vi "Mask Joysticks.vi"(6 "Operator POVs":i16[](array[numeric])=[-1], 7 "Driver Axes":dbl[](array[numeric]), 8 "Operator Buttons":bool[](array[boolean])=[FALSE, FALSE, FALSE, FALSE, FALSE, FALSE, FALSE, FALSE, FALSE, FALSE], 9 "Operator Axes":dbl[](array[numeric])=[0.0, -0.007874015748031496, 0.0, 0.0, 0.0, 0.0], 10 "Driver POVs":i16[](array[numeric]), 11 "Driver Buttons":bool[](array[boolean])=[TRUE, FALSE, FALSE, FALSE, FALSE, FALSE, FALSE, FALSE, FALSE, TRUE]) -> (0 "Operator Buttons Out":bool[](array[boolean]), 1 "Operator Axes Out":dbl[](array[numeric]), 2 "Driver POVs Out":i16[](array[numeric]), 3 "Drive Buttons Out":bool[](array[boolean])=[TRUE, FALSE, FALSE, FALSE, FALSE, FALSE, FALSE, FALSE, FALSE, TRUE], 4 "Operator POVs Out":i16[](array[numeric])=[-1], 5 "Drive Axes Out":dbl[](array[numeric]))   [LabVIEW 2018]
panel:
  out "Time to excecute ms":u32
  in  "Operator Axes Mask":bool[](array[boolean])=[TRUE, TRUE, TRUE, TRUE, TRUE, TRUE, TRUE, TRUE, TRUE, TRUE]
  in  "Operator Buttons Mask":bool[](array[boolean])=[TRUE, TRUE, TRUE, TRUE, TRUE, TRUE, TRUE, TRUE, TRUE, TRUE]
  in  "D315":bool
  in  "D270":bool
  in  "D235":bool
  in  "D135":bool
  in  "D180":bool
  in  "D90":bool
  in  "D45":bool
  in  "D0/360":bool
  in  "Driver Buttons Mask":bool[](array[boolean])=[TRUE, TRUE, TRUE, TRUE, TRUE, TRUE, TRUE, TRUE, TRUE, TRUE]
  in  "Driver Axes Mask":bool[](array[boolean])=[TRUE, TRUE, TRUE, TRUE, TRUE, TRUE, TRUE, TRUE, TRUE, TRUE]
  # "POV Mask"
  # "POV Masking Not DOne"
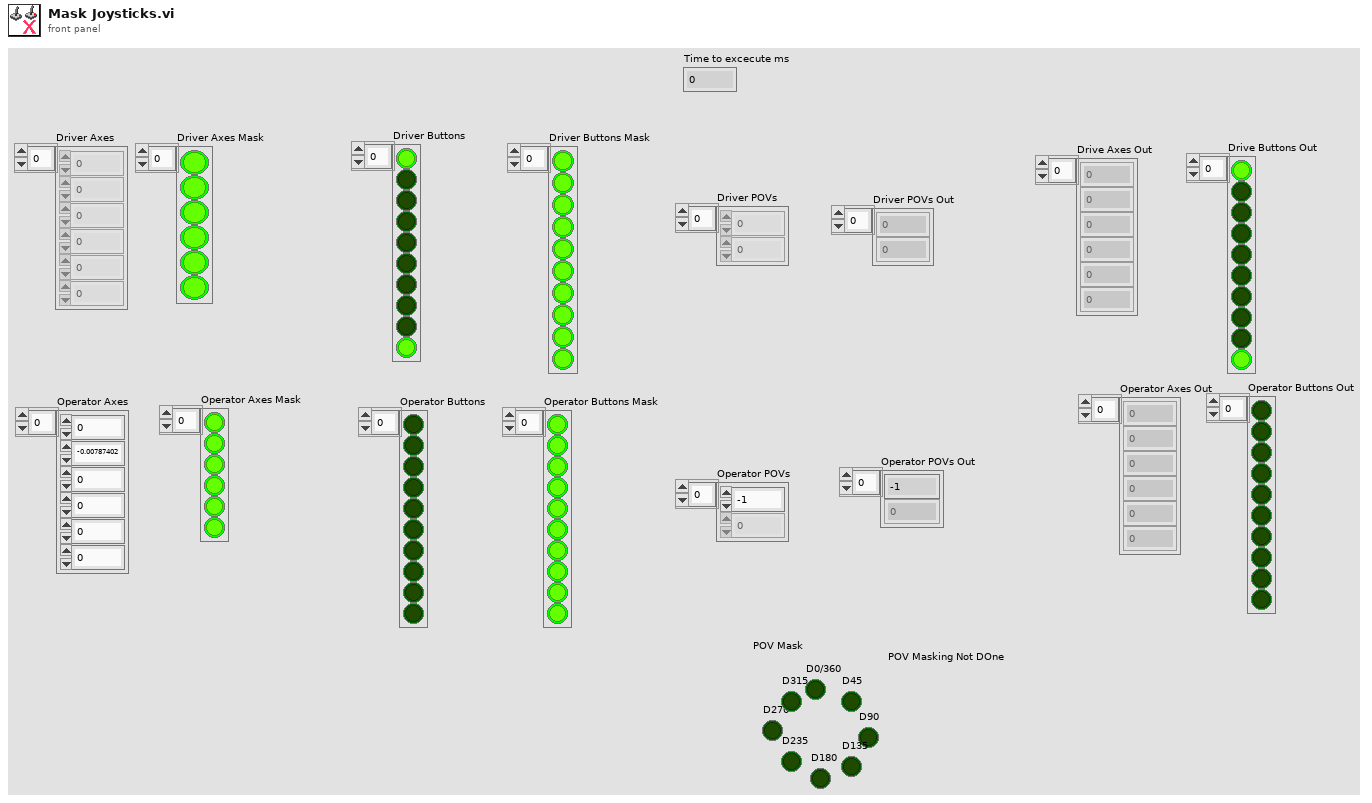
[diagram p1: front panel]
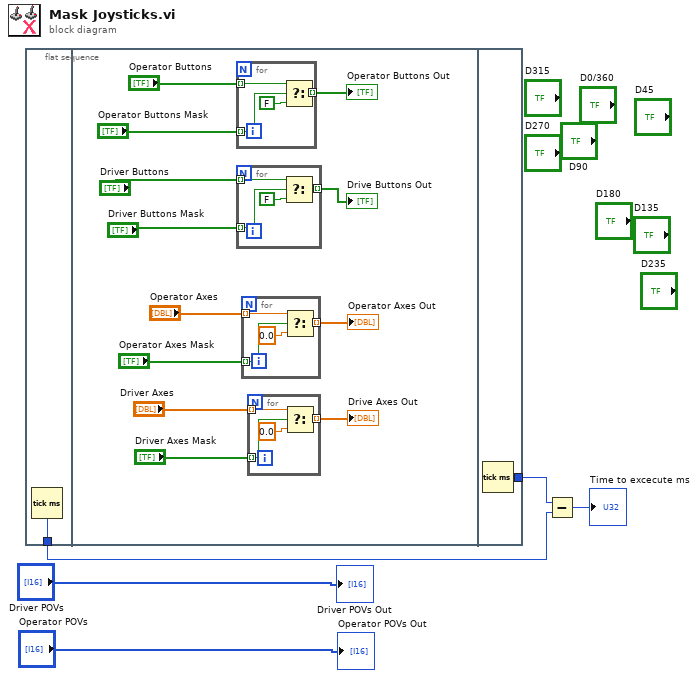
[diagram p0: block diagram]
diagram:
  n1 = flat-sequence {
    tunnel: [w6] -> w2
    tunnel: [w35] -> w3
    frame #0 {
      n2 = Tick Count (ms)() -> (millisecond timer value=w6:u32)
    }
    frame #1 {
      n3 = for {
        tunnel: [w34] -> w16 mode=indexing
        tunnel: "Operator Buttons Mask" -> [w33] mode=indexing
        tunnel: "Operator Buttons" -> [w32] mode=indexing
        n4 = Select(t=w32, s=w33, f=FALSE) -> (s? t:f=w34:bool)
      }
      "Operator Buttons Out" <- w16
      n5 = for {
        tunnel: "Driver Buttons Mask" -> [w30] mode=indexing
        tunnel: "Driver Buttons" -> [w29] mode=indexing
        tunnel: [w28] -> w17 mode=indexing
        n6 = Select(t=w29, s=w30, f=FALSE) -> (s? t:f=w28:bool)
      }
      "Drive Buttons Out" <- w17
      n7 = for {
        tunnel: [w26] -> w14 mode=indexing
        tunnel: "Operator Axes Mask" -> [w25] mode=indexing
        tunnel: "Operator Axes" -> [w24] mode=indexing
        n8 = Select(t=w24, s=w25, f=0.0) -> (s? t:f=w26:dbl)
      }
      "Operator Axes Out" <- w14
      n9 = for {
        tunnel: [w22] -> w13 mode=indexing
        tunnel: "Driver Axes" -> [w21] mode=indexing
        tunnel: "Driver Axes Mask" -> [w20] mode=indexing
        n10 = Select(t=w21, s=w20, f=0.0) -> (s? t:f=w22:dbl)
      }
      "Drive Axes Out" <- w13
    }
    frame #2 {
      n11 = Tick Count (ms)() -> (millisecond timer value=w35:u32)
    }
  }
  n12 = Subtract(x=w3, y=w2) -> (x-y=→"Time to excecute ms":u32)
  "Driver POVs Out" <- "Driver POVs"
  "Operator POVs Out" <- "Operator POVs"
